vi "Find All Character.vi"(9 "Character":string, 11 "Input String":string) -> (1 "Number":i32, 2 "Strings":string[](array[string]), 3 "Indicies":i32[](array[numeric]))   [LabVIEW 2017]
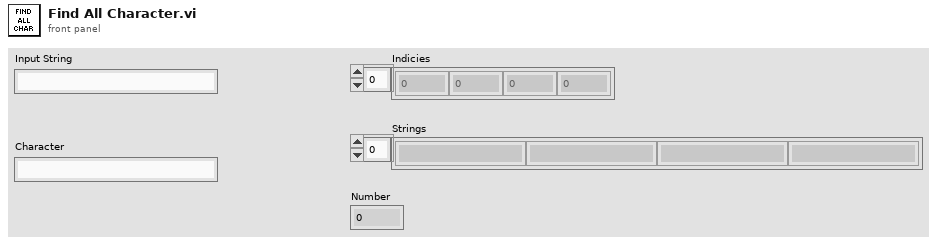
[diagram p1: front panel]
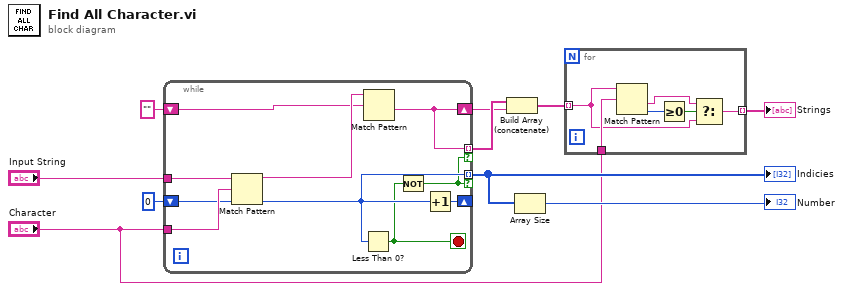
[diagram p0: block diagram]
diagram:
  n1 = while {
    tunnel: "Input String" -> [w20]
    tunnel: "Character" -> [w19]
    shift-right: [w17] -> _
    shift-left: 0 ("offset past match") -> [w18]
    tunnel: [w16] -> w8 mode=indexing if=w14
    tunnel: [w11] -> w6 mode=indexing if=w14
    shift-right: [w11] -> w4
    shift-left: "" ("Input String") -> [w12]
    stop <- w15 stop-if-true
    n2 = Match Pattern(string=w20, regular expression=w19, offset (0)=w18) -> (before substring=w13:string, offset past match=w16:i32)  [unwired: 2 out]
    n3 = Less Than 0?(x=w16) -> (x < 0?=w15:bool)
    n4 = Match Pattern(string=w13, regular expression=w12) -> (after substring=w11:string)  [unwired: 1 in, 3 out]
    n5 = Not(x=w15) -> (.not. x?=w14:bool)
    n6 = Increment(x=w16) -> (x+1=w17:i32)
  }
  "Indicies" <- w8
  n7 = Build Array (concatenate)(w6, w4) -> (w3:string[])
  n8 = Array Size(array=w8) -> (size(s)=→"Number":i32)
  n9 = for {
    tunnel: w3 -> [w22] mode=indexing
    tunnel: "Character" -> [w26]
    tunnel: [w21] -> w1 mode=indexing
    n10 = Match Pattern(string=w22, regular expression=w26) -> (after substring=w23:string, offset past match=w25:i32)  [unwired: 1 in, 2 out]
    n11 = Greater Or Equal To 0?(x=w25) -> (x >= 0?=w24:bool)
    n12 = Select(t=w23, s=w24, f=w22) -> (s? t:f=w21:string)
  }
  "Strings" <- w1
